vi "average.vi"(1 "Array":dbl[](array[numeric])) -> (0 "Average":dbl)   [LabVIEW 2017]
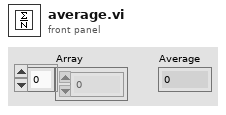
[diagram p1: front panel]
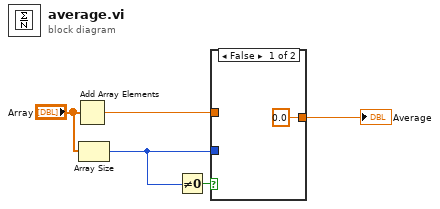
[diagram p0: block diagram]
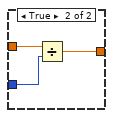
[diagram p2: hidden frame]
diagram:
  n1 = Add Array Elements(numeric array="Array") -> (sum=w3:dbl)
  n2 = Array Size(array="Array") -> (size(s)=w1:i32)
  n3 = Not Equal To 0?(x=w1) -> (x != 0?=w2:bool)
  n4 = case shown="False" w2 {
    tunnel: [0.0 w9] -> w5
    tunnel: w1 -> [_ w8]
    tunnel: w3 -> [_ w7]
    frame False {
    }
    frame True {
      n5 = Divide(x=w7, y=w8) -> (x/y=w9:dbl)
    }
  }
  "Average" <- w5
